vi "Get Invalid Scalar Data Channels.vi"(8 "error in (no error)":errorcluster, 10 "new bitfile scalar channels":T4[](array[typedef]) {"Data Type" format="%.0x"}, 11 "old bitfile scalar channels":T1[](array[typedef]) {"Item Ref" format="%.0x"}) -> (0 "error out":errorcluster, 2 "valid scalar channels":T1[](array[typedef]) {"Item Ref" format="%.0x"}, 3 "invalid scalar channels":T1[](array[typedef]) {"Item Ref" format="%.0x"})   [LabVIEW 2019, in "FPGA Addon System Explorer.lvlib"]
uses:
  FPGA Addon System Explorer.lvlib
  Addon Shared/Types/Register Information.ctl
  Addon Shared/Types/FPGA Addon Data Type.ctl
  Types/Output Scalar.ctl
  <vilib>/NI VeriStand/Custom Device API/Custom Device Item Ref.ctl
  Addon Shared/FPGA Addon Shared.lvlib
  <vilib>/NI VeriStand/Custom Device API/Custom Device API.lvlib
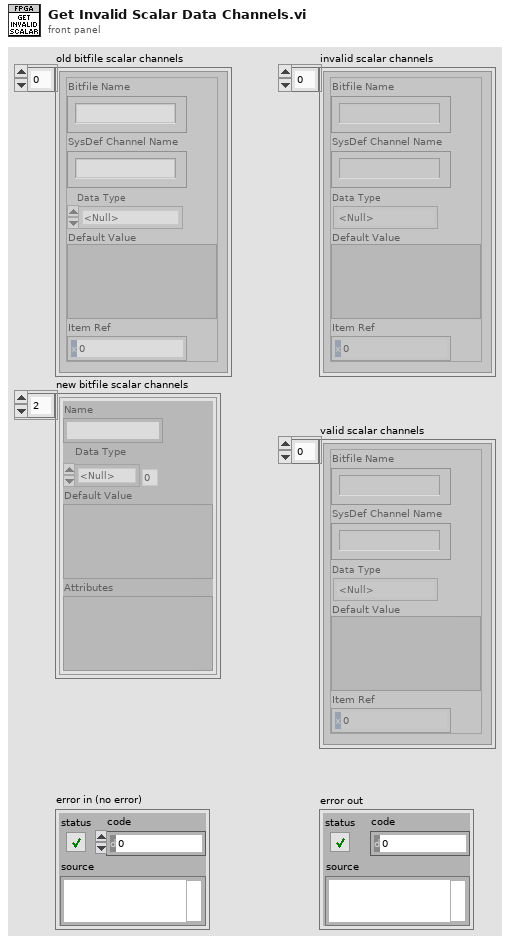
[diagram p1: front panel]
types:
  T1 = typedef "FPGA Addon System Explorer.lvlib/Output Scalar.ctl" = cluster{"Bitfile Name":string, "SysDef Channel Name":string, "Data Type":T2, "Default Value":variant, "Item Ref":T3}
  T2 = typedef "FPGA Addon Shared.lvlib/FPGA Addon Data Type.ctl" = enum8{"<Null>", "I8", "I16", "I32", "I64", "U8", "U16", "U32", "U64", "SGL", "Boolean", "Analog PWM In Settings", "Analog PWM In", "Digital PWM In Settings", "Digital PWM In", "Digital PWM Out", "Sine Out", "FXP", "FXP+/-24.5", "FXP+/-16.5", "FXP+/-32.8", "FXP+/-64.32", "FXP+/-16.7", "FXP+/-20.5", "FXP+/-27.5", "FXP+/-32.16", "FXP+16.3", "FXP+18.3", "Digital Static In", "Digital Static Out", "Digital Static In Settings", "Digital WSS Out", "Quad Encoder Settings", "Quad Encoder In", "Group"}
  T3 = typedef "Custom Device API.lvlib/Custom Device Item Ref.ctl" = u64
  T4 = typedef "FPGA Addon Shared.lvlib/Register Information.ctl" = cluster{"Name":string, "Data Type":T2, "Default Value":variant, "Attributes":variant}
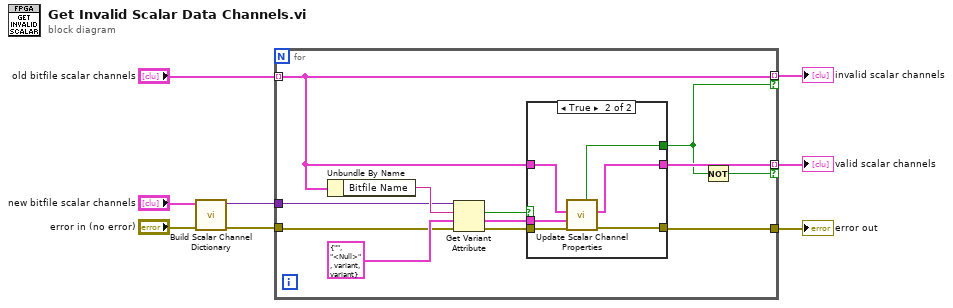
[diagram p0: block diagram]
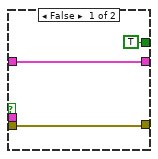
[diagram p2: hidden frame]
diagram:
  n1 = call "Build Scalar Channel Dictionary.vi"("error in (no error)"="error in (no error)", "scalar channels"="new bitfile scalar channels") -> ("error out"=w3:errorcluster, "scalar channels dictionary"=w2:variant)  [unwired: 8 in]
  n2 = for {
    tunnel: [w20] -> w6
    tunnel: "old bitfile scalar channels" -> [w18] mode=indexing
    tunnel: [w18] -> w4 mode=indexing if=w10
    tunnel: w3 -> [w15]
    tunnel: w2 -> [w14]
    tunnel: [w19] -> w1 mode=indexing if=w9
    n3 = Unbundle By Name(w18) -> ("Bitfile Name"=w17:string)
    n4 = Get Variant Attribute(Variant=w14, name=w17, default value (empty Variant)=T4 {"Name"="", "Data Type"=enum."<Null>", "Default Value"=variant, "Attributes"=variant}, error in=w15) -> (found=w13:bool, value=w11:T4, error out=w12:errorcluster)  [unwired: 1 out]
    n5 = case shown="True" w13 {
      tunnel: w18 -> [w21 w26]
      tunnel: [w22 w29] -> w20
      tunnel: [TRUE w24] -> w10
      tunnel: [w21 w28] -> w19
      tunnel: w12 -> [w22 w27]
      tunnel: w11 -> [_ w25]
      frame False {
      }
      frame True {
        n6 = call "Update Scalar Channel Properties.vi"("error in (no error)"=w27, "new bitfile scalar channel"=w25, "old bitfile scalar channel"=w26) -> ("error out"=w29:errorcluster, "scalar channel out"=w28:T1, "remove"=w24:bool)  [unwired: 6 in]
      }
    }
    n7 = Not(x=w10) -> (.not. x?=w9:bool)
  }
  "error out" <- w6
  "invalid scalar channels" <- w4
  "valid scalar channels" <- w1
